vi "DSF.Engine.Runtime.Framework.Set Sequencer.vi"(8 "error in (no error)":errorcluster, 10 "Sequencer":refnum<class "DSF.Engine.Sequencer.lvclass">, 11 "Framework Runtime in":refnum<class "DSF.Engine.Runtime.Framework.lvclass">) -> (0 "error out":errorcluster, 3 "Framework Runtime out":refnum<class "DSF.Engine.Runtime.Framework.lvclass">)   [LabVIEW 2017, in "DSF.Engine.lvlib" / "DSF.Engine.Runtime.Framework.lvclass"]
uses:
  DSF.Engine.Runtime.Framework.lvclass
  Sequencer/DSF.Engine.Sequencer.lvclass
  DSF.Engine.Runtime.Framework.lvclass/DSF.Engine.Runtime.Framework.ctl
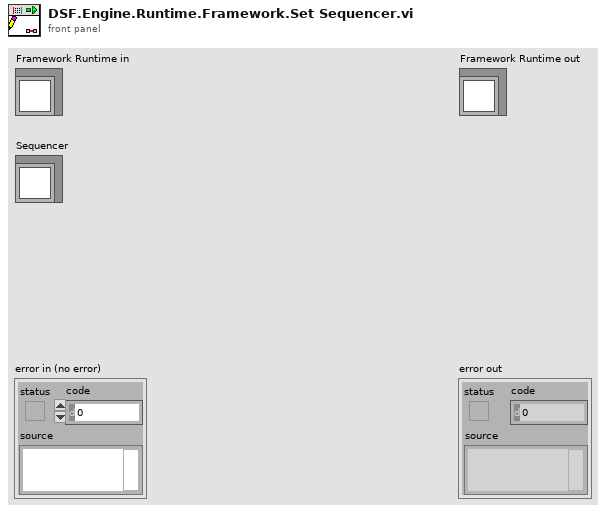
[diagram p1: front panel]
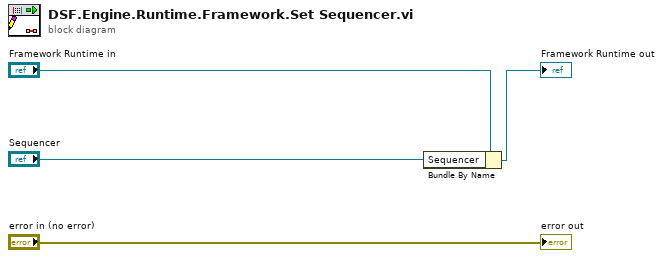
[diagram p0: block diagram]
diagram:
  n1 = Bundle By Name(cluster="Framework Runtime in", "Sequencer"="Sequencer") -> (→"Framework Runtime out":refnum<class "DSF.Engine.Runtime.Framework.lvclass">)
  "error out" <- "error in (no error)"
